vi "Get BLISS_Username and PW PG.vi"() -> (0 "error out":errorcluster, 2 "Password Out":string="Magyar09", 3 "User Name Out":string="varga.sm@pg.com")   [LabVIEW 2020]
uses:
  Get BLISS_Global Error Codes.vi
panel:
  in  "OK":bool=TRUE
  in  "Password":string
  in  "User Name":string="@pg.com"
  # "BLISS Server Access"
  # "https://itaccess.pg.com/identityiq/ui/external/desktopResetUsername.jsf"
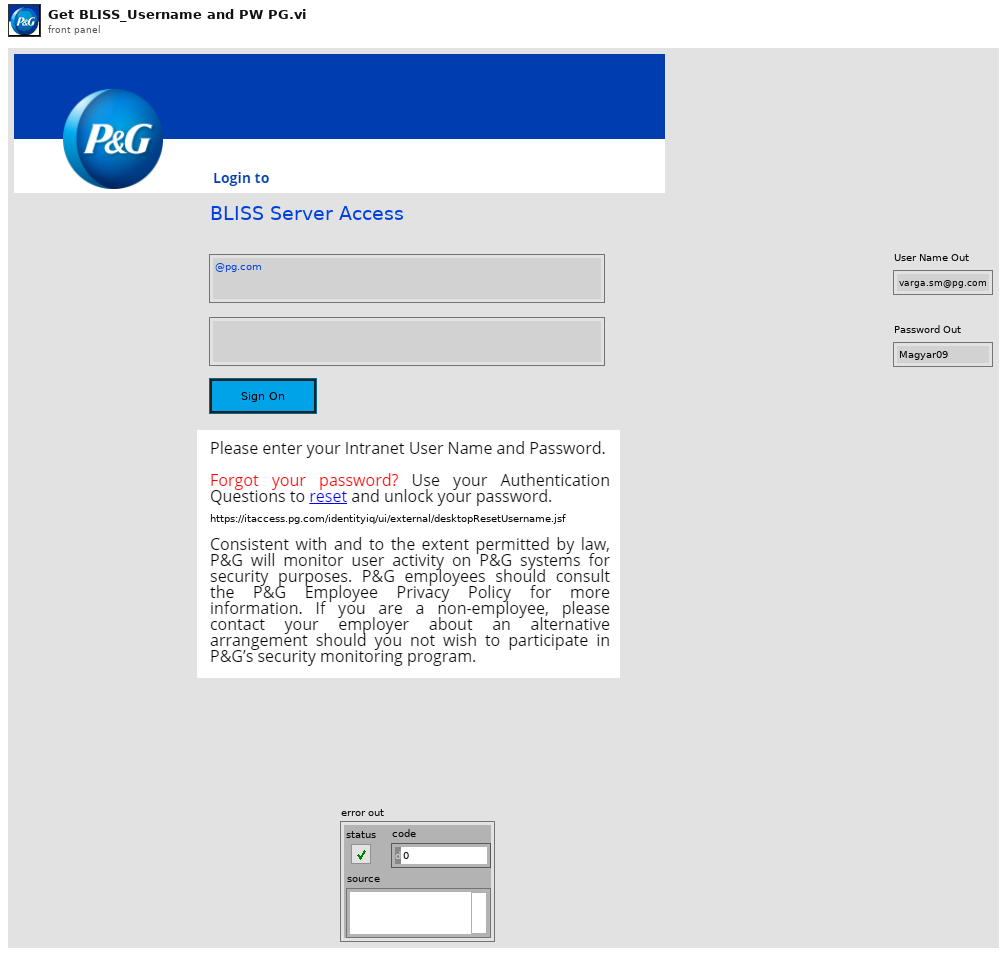
[diagram p1: front panel]
types:
  T1 = typedef "eventvkey.ctl" = enum16{"ASCII", "Enter", "Return", "Shift", "Ctrl", "Alt", "Cmd", "Opt", "Caps", "NumLock", "Clear", "Break", "Up", "Down", "Left", "Right", "Insert", "Delete", "Home", "End", "PageUp", "PageDown", "Escape", "Help", "Pause", "ScrollLock", "F1", "F2", "F3", "F4", "F5", "F6", "F7", "F8", "F9", "F10", "F11", "F12", "F13", "F14", "F15", "F16", "F17", "F18", "F19", "F20", "F21", "F22", "F23", "F24", "Play", "VolumeUp", "VolumeDown", "Mute", "Two Byte Char"}
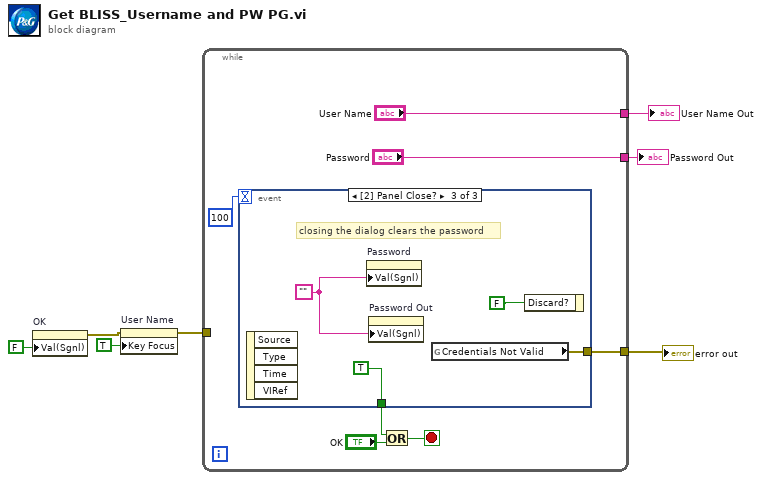
[diagram p0: block diagram]
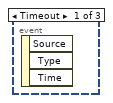
[diagram p2: hidden frame]
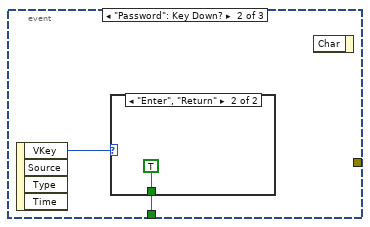
[diagram p3: hidden frame]
diagram:
  n1 = property on="OK" class="Bool (strict)"("Val(Sgnl)"=FALSE ("Value (Signaling)")) -> (error out=w2:errorcluster)  [unwired: 2 in, 1 out]
  n2 = property on="User Name" class="Str"(error in=w2, "Key Focus"=TRUE) -> (error out=w4:errorcluster)  [unwired: 1 in, 1 out]
  n3 = while {
    tunnel: ["User Name"] -> w6
    tunnel: ["Password"] -> w5
    tunnel: w4 -> [_]
    tunnel: [w8] -> w1
    stop <- w12 stop-if-true
    n4 = event shown="[2] Panel Close?" {
      selector: _ -> [_ _ _]
      dyn-events: _ -> [_ _ _]
      timeout: 100 -> [_ _ _]
      tunnel: [_ w16 TRUE] -> w11
      tunnel: [_ _ w18] -> w8
      event Timeout {
        n5 = event-data() -> ()  [unwired: 1 in, 3 out]
      }
      event "Password": Key Down? {
        n6 = event-data() -> ("VKey"=w15:T1)  [unwired: 1 in, 3 out]
        n7 = case shown="\"Enter\", \"Return\"" w15 {
          tunnel: [_ TRUE] -> w16
          frame "ASCII", Default {
          }
          frame "Enter", "Return" {
          }
        }
        n8 = event-data() -> ()  [unwired: 2 in, 1 out]
      }
      event Panel Close? {
        w21 = ""
        # "closing the dialog clears the password"
        n9 = event-data() -> ()  [unwired: 1 in, 4 out]
        n10 = property on="Password" class="Str"("Val(Sgnl)"=w21) -> ()  [unwired: 2 in, 2 out]
        n11 = property on="Password Out" class="Str"("Val(Sgnl)"=w21) -> ()  [unwired: 2 in, 2 out]
        n12 = global read "Get BLISS_Global Error Codes.vi" "Credentials Not Valid"() -> (w18:errorcluster)
        n13 = event-data("Discard?"=FALSE) -> ()  [unwired: 1 in, 1 out]
      }
    }
    n14 = Or(x=w11, y="OK") -> (x .or. y?=w12:bool)
  }
  "User Name Out" <- w6
  "Password Out" <- w5
  "error out" <- w1
